vi "SVA 4MV6 P01 CCE RRMA.vi"() -> ()   [LabVIEW 2020]
doc: "Ceballos Conde Emanuel Rodríguez Ramírez Miguel Ángel 4MV6 Sistemas de visión artificial 2022/1\nEste vi permite obtener la distancia en X y Z a la cual se encuentra en objeto u objetos(un maximo de 3 siempre y cuando el color de cada objeto sea de cada una las componentes del sistema rgb) de un sisitema de vision estereoscopico. el usuario puede definir el foco y la distancia del sisitema, a su vez presenta las capturas obtenidas de dichas camara, una representacion en 3d (en el plano XZ) de la escena capturada y permite observar la imagenes binarizadas obtenidas de la descomosicion rgb de cada captura"
uses:
  <vilib>/userDefined/High Color/IMAQdx.ctl
  SVA 4MV6 P01 CCE RRMA.ctl
  <vilib>/vision/driver/IMAQdx.llb/IMAQdx Buffer Number Mode.ctl
  <vilib>/vision/driver/NI_Vision_Acquisition_Software.lvlib
panel:
  in  "umbral\nsuperior":u8=255
  in  "umbral\ninferior":u8=100
  out "Espera":bool
  out "Escena recreada":refnum<vi>(3d-picture)
  in  "Foco\nde la \ncamara":dbl=1331.0
  in  "Distancia\nentre \ncamaras":dbl=20.0 format="%#_13g"
  out "XR":i32
  out "XB":i32
  out "XG":i32
  out "Imagen binaria azul  izquierda":T1(plugin-control)
  out "Imagen binaria verde  izquierda":T1(plugin-control)
  out "Imagen binaria roja  izquierda":T1(plugin-control)
  out "Imagen binaria azul  derecha":T1(plugin-control)
  out "Imagen binaria verde derecha":T1(plugin-control)
  out "Imagen binaria roja  derecha":T1(plugin-control)
  out "ZB":i32
  out "ZG":i32
  out "ZR":i32
  out "Cal Dis":bool
  out "Cap izq":bool
  out "Cap der":bool
  in  "calcular distancia":bool
  in  "capturar imagen izquierda":bool
  in  "capturar Imagen derecha":bool
  out "Imagen izquierda":T1(plugin-control)
  out "Entrada de video":T1(plugin-control)
  in  "stop":bool
  in  "Session In":T2
  out "Imagen derecha":T1(plugin-control)
  # "Controles"
  # "Ceballos Conde Emanuel\nRodríguez Ramírez Miguel Ángel\n4MV6\nSistemas de visión artificial\n2022/1"
  # "Estado"
  # "Resultados en cm"
  # "Configuración"
  # "Binarizado"
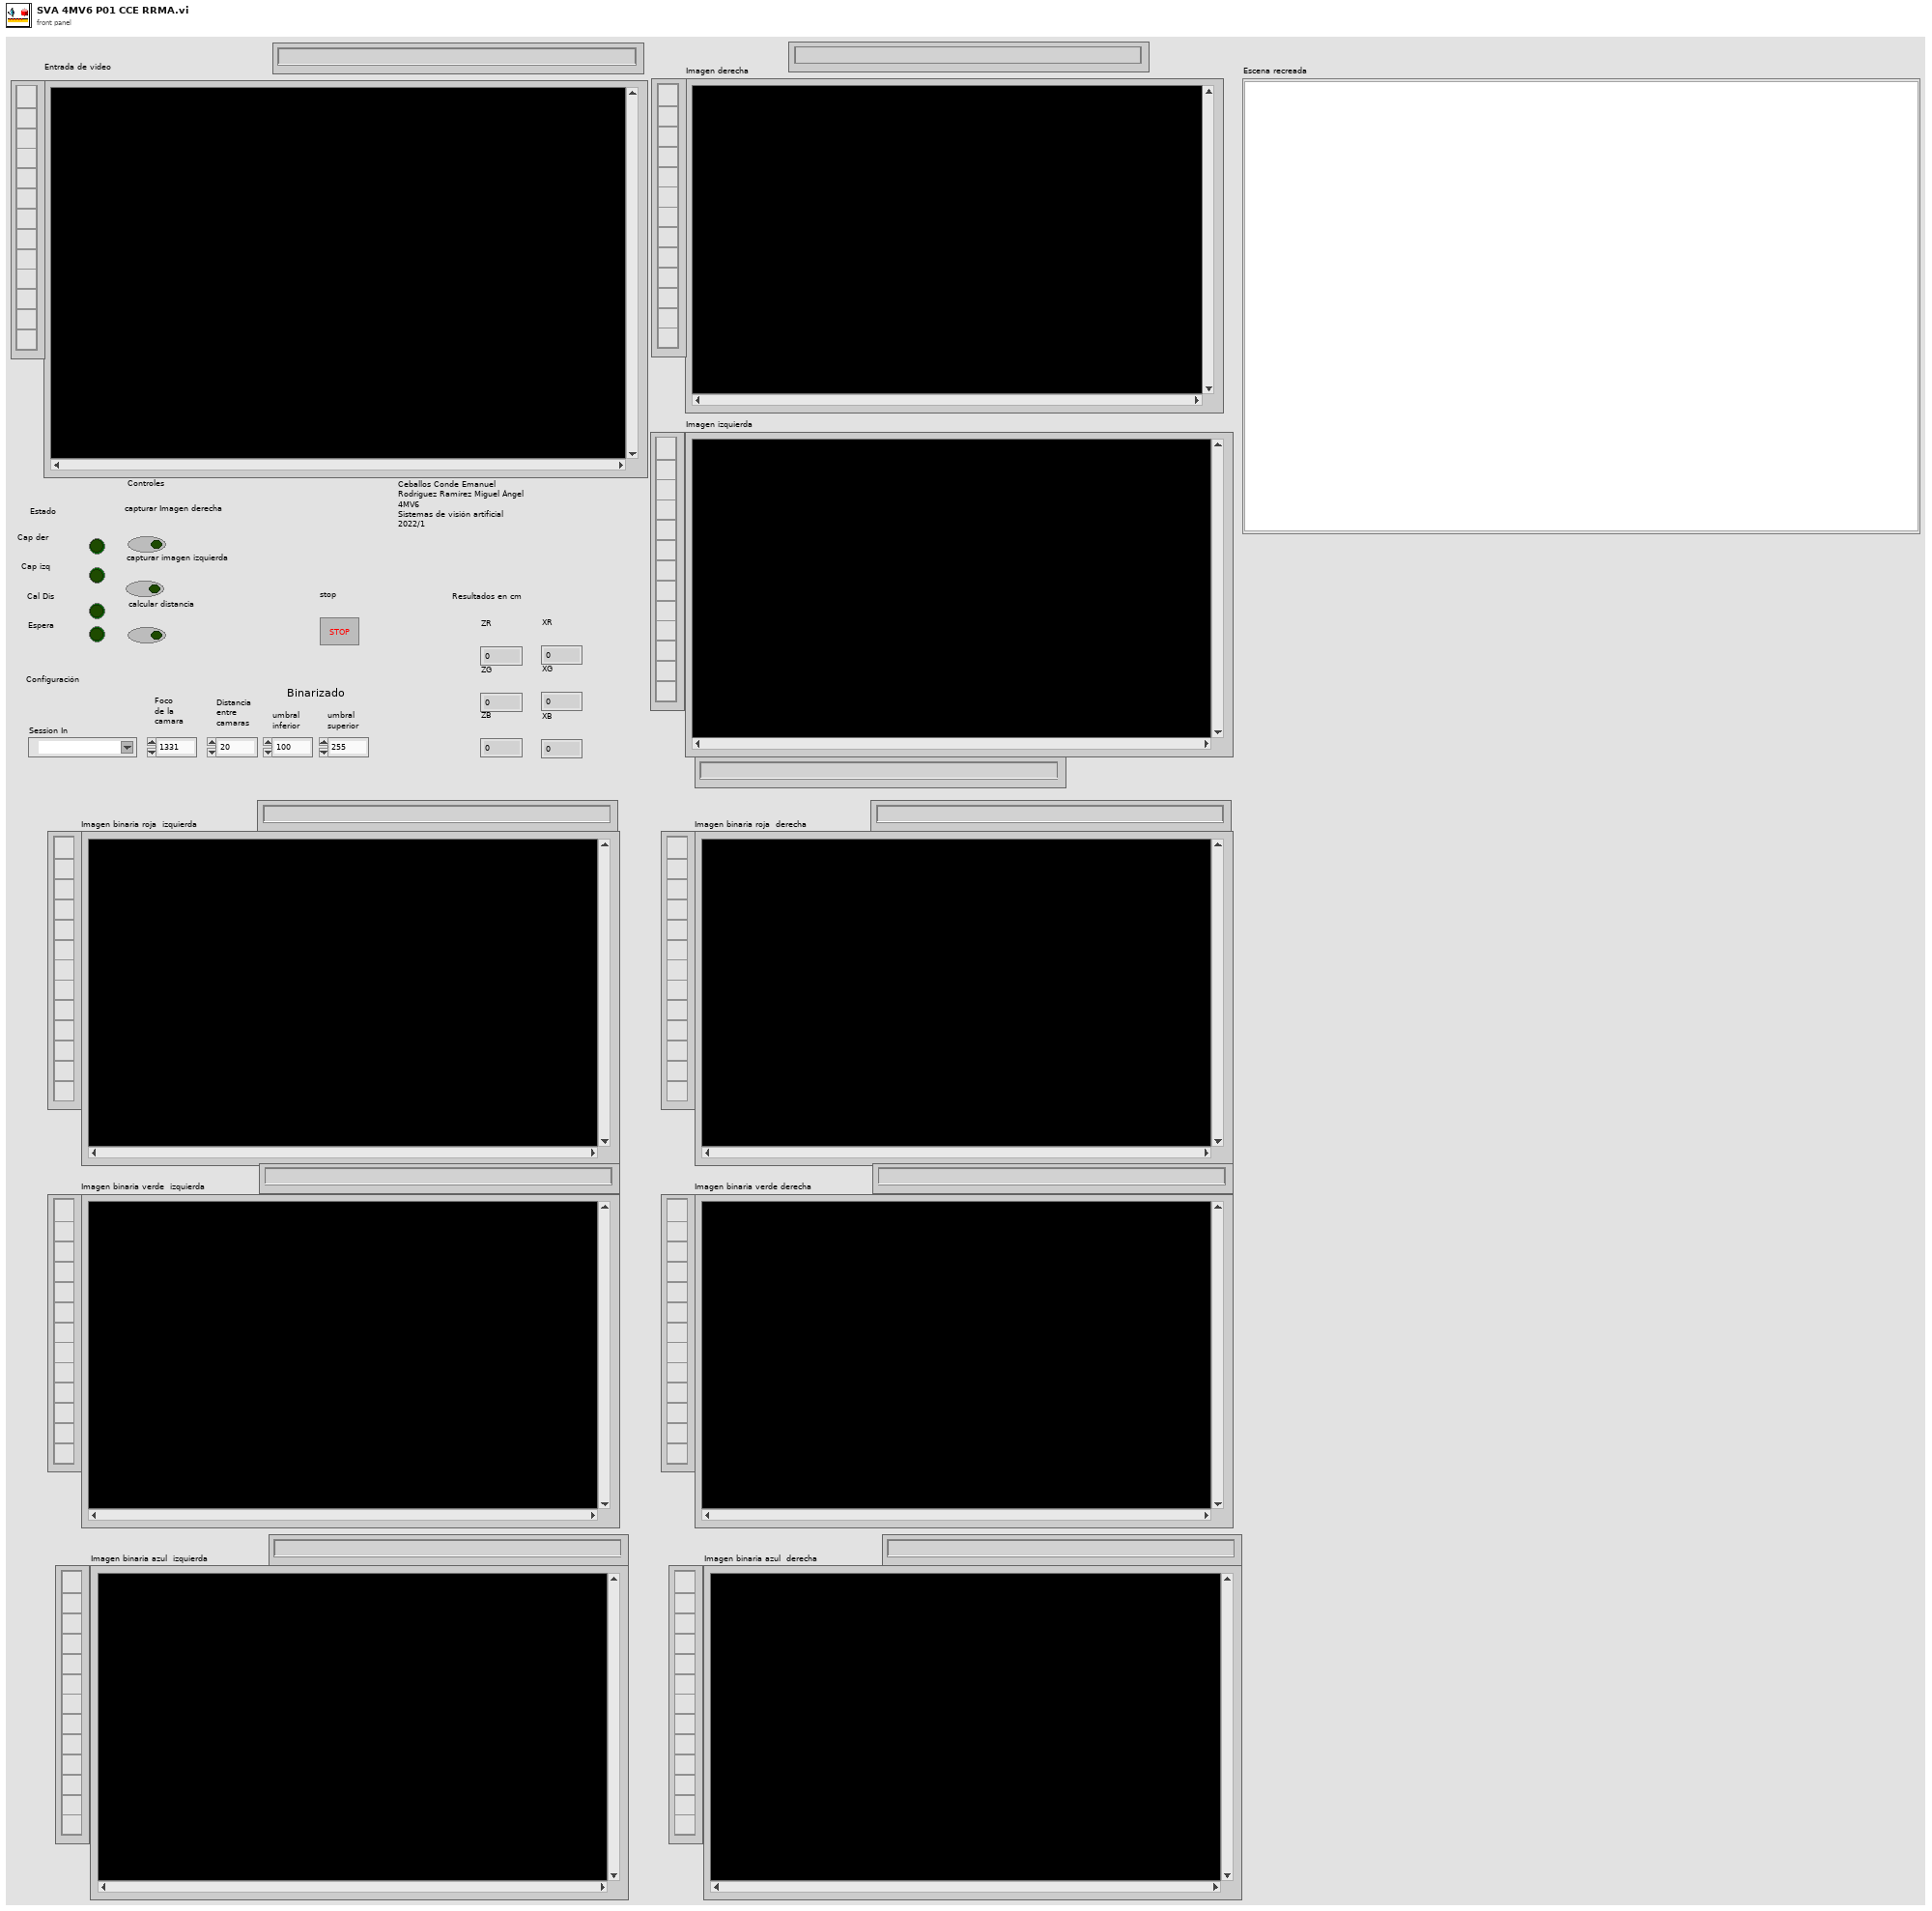
[diagram p1: front panel]
types:
  T1 = typedef "IMAQ Image.ctl" = refnum<image>
  T2 = typedef "IMAQdx.ctl" = refnum<k21>
  T3 = typedef "Image Type" = u32
  T4 = typedef "SVA 4MV6 P01 CCE RRMA.ctl" = enum16{"captura imagen derecha", "captura imagen izquierda", "calculo de distancia", "espera"}
  T5 = typedef "NI_Vision_Acquisition_Software.lvlib/IMAQdx Buffer Number Mode.ctl" = enum32{"Next", "Last", "Buffer Number", "Every", "Last New"}
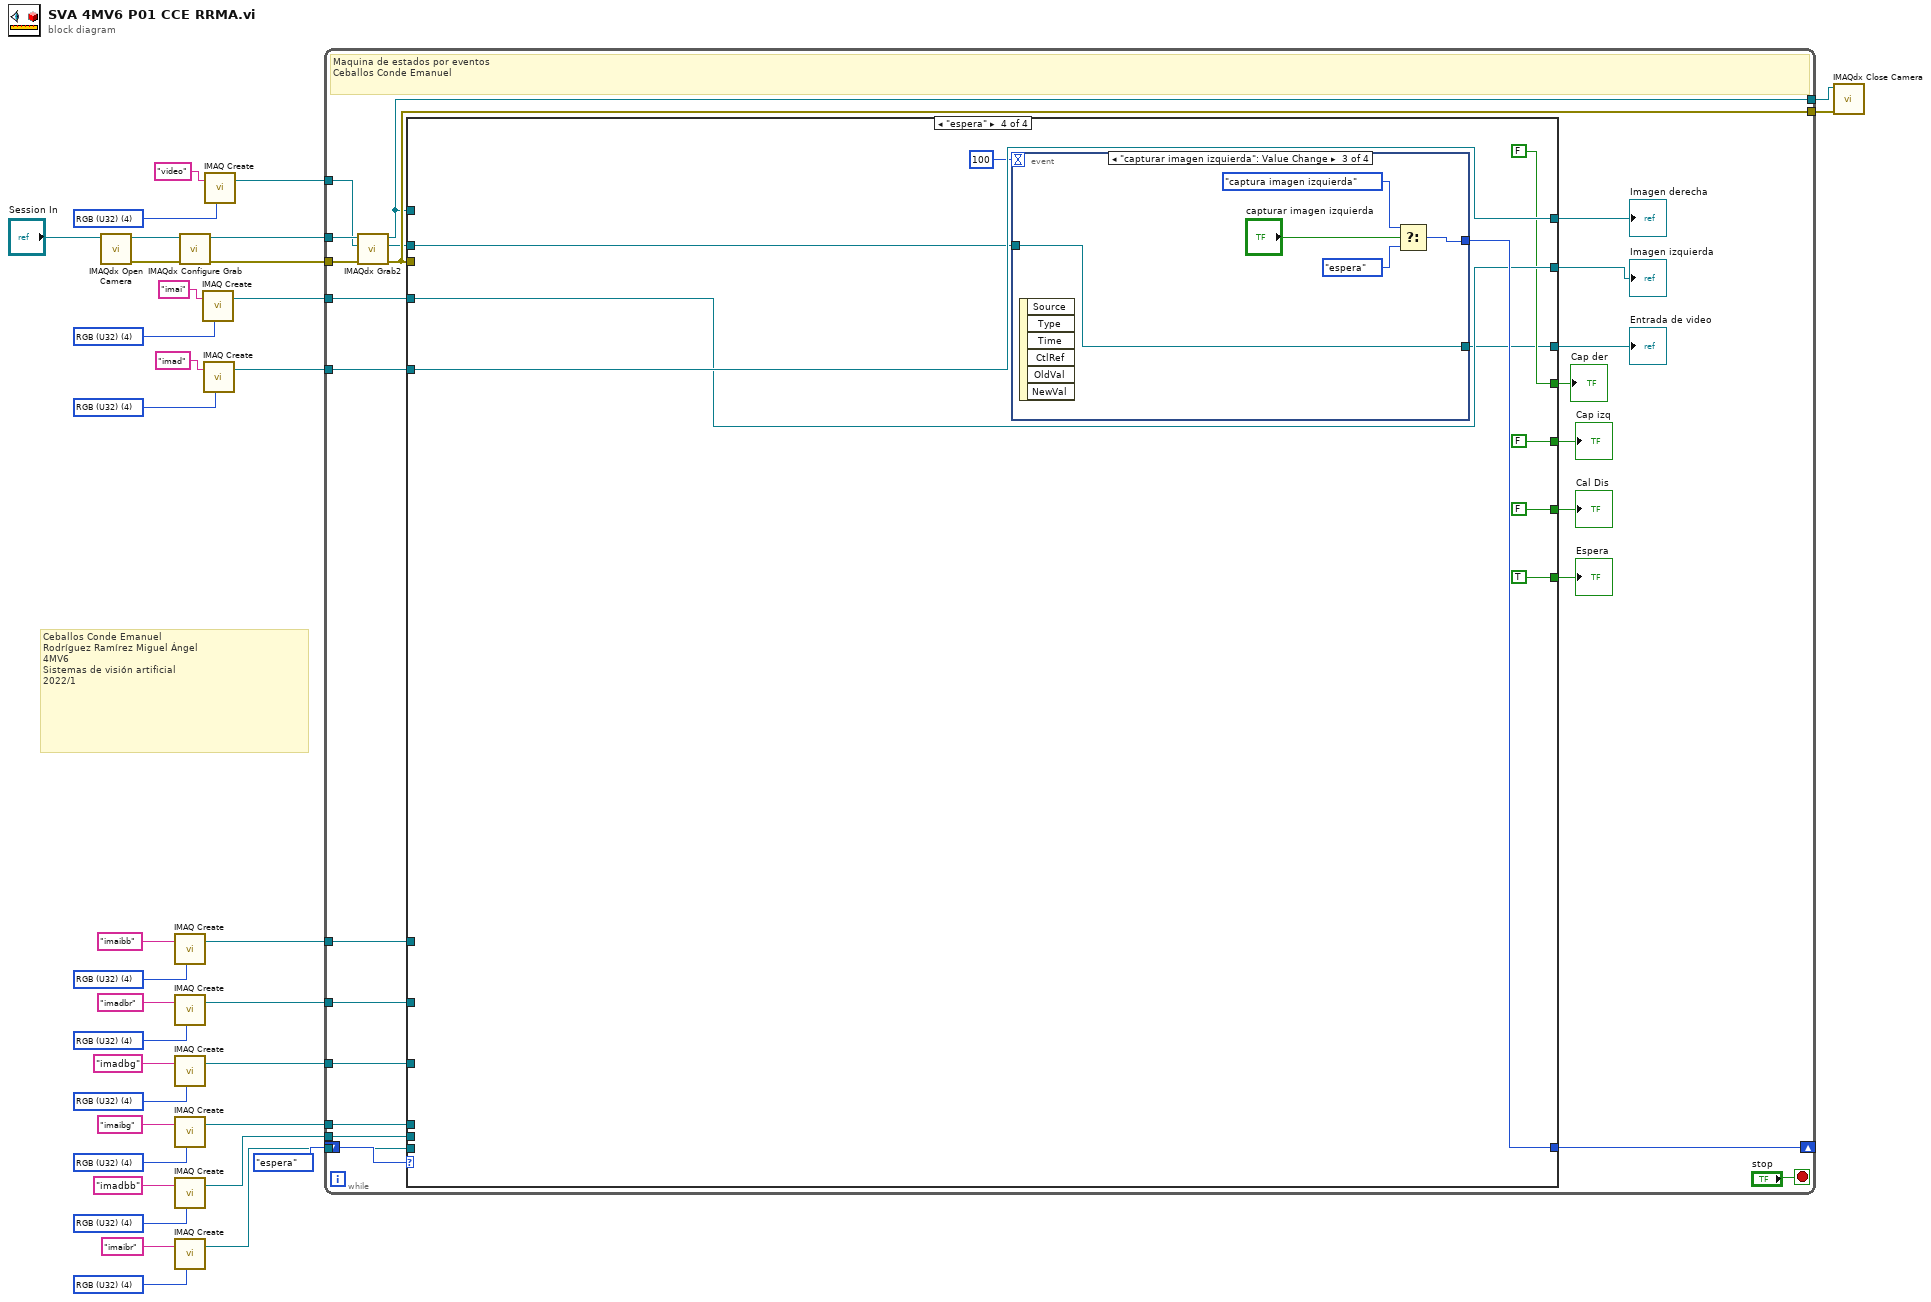
[diagram p0: block diagram]
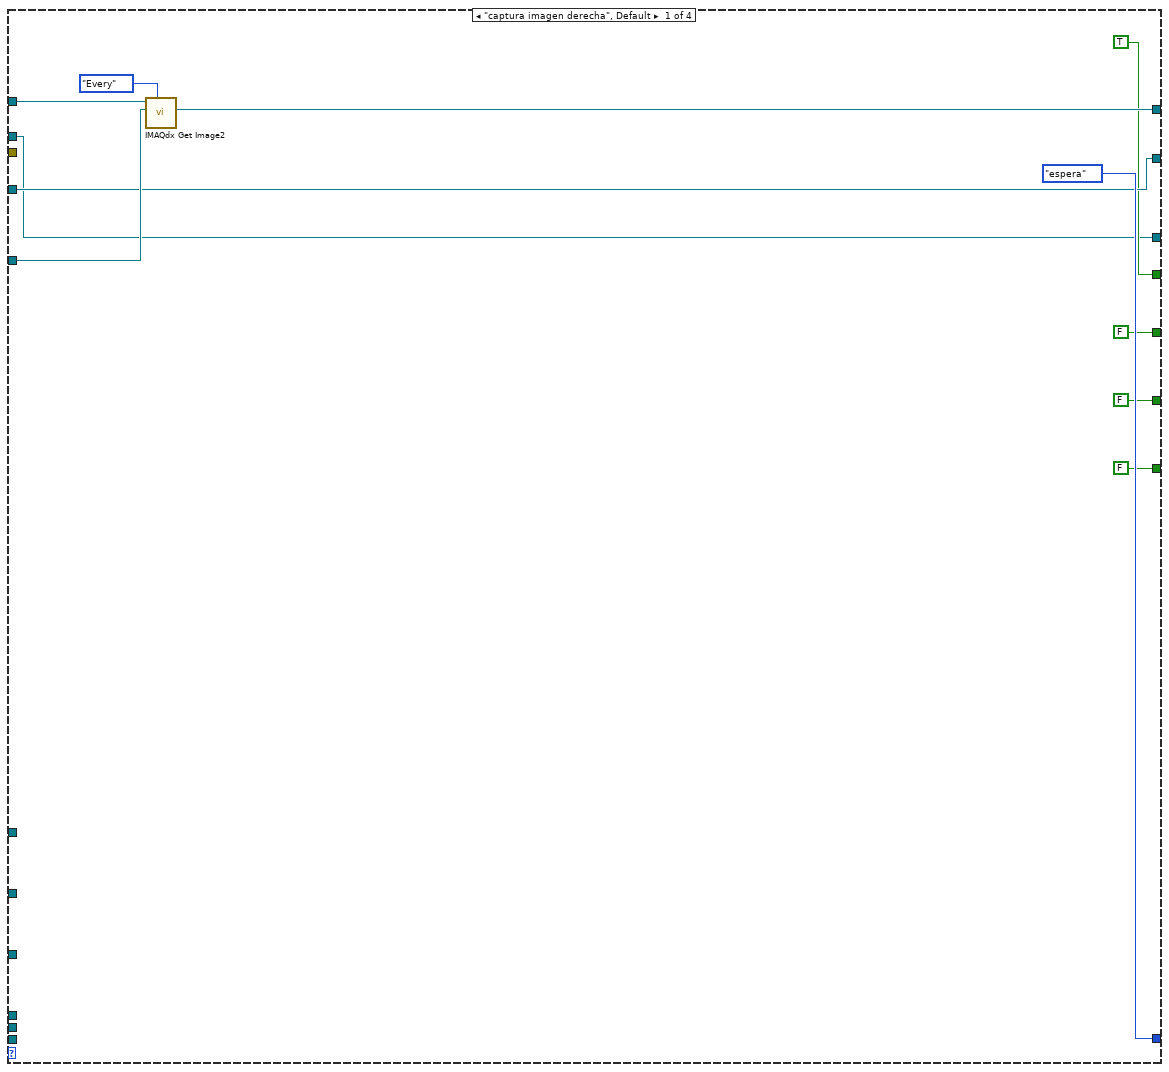
[diagram p2: hidden frame]
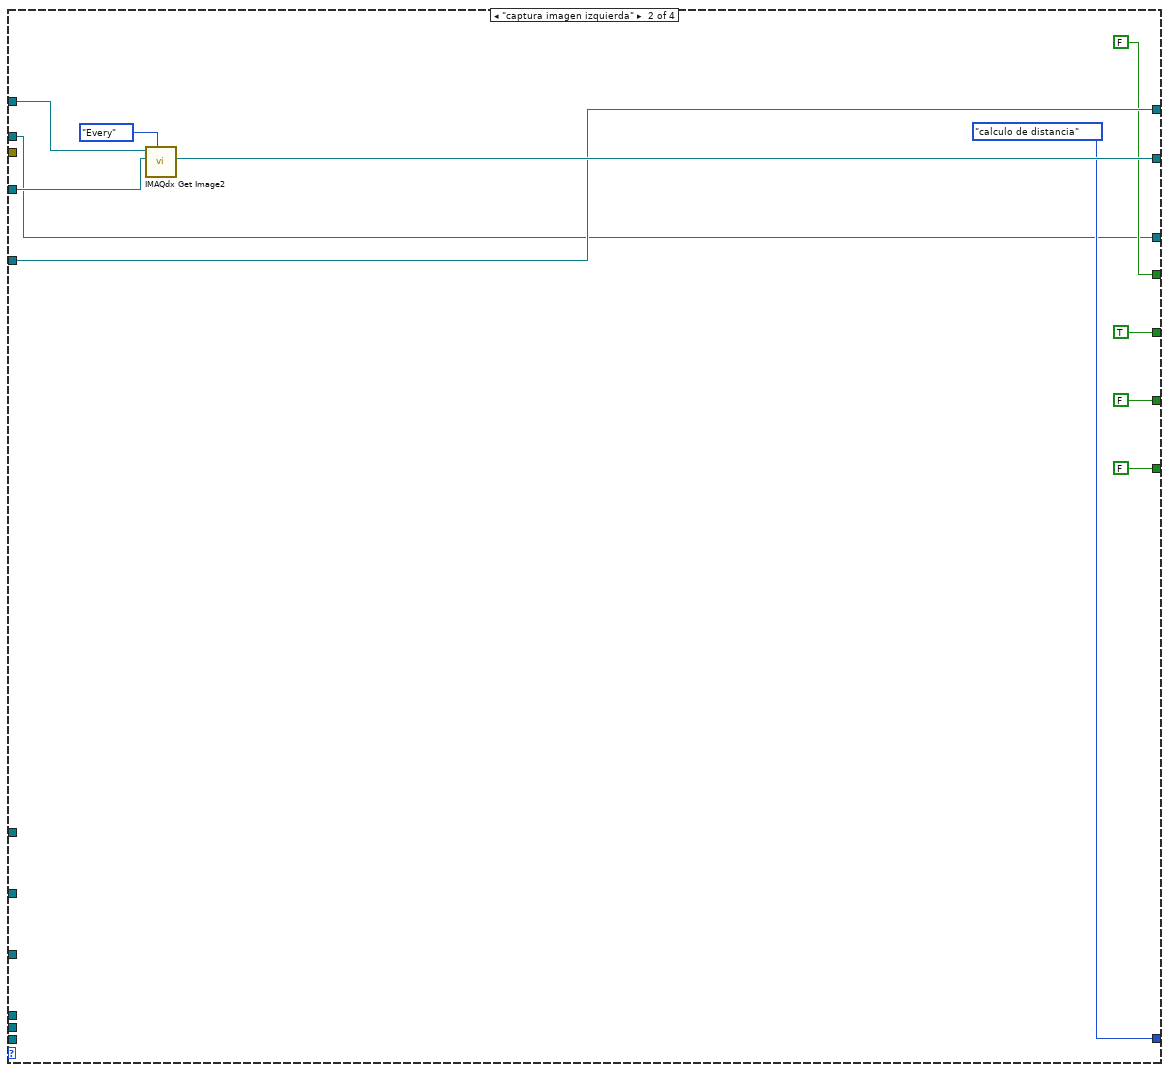
[diagram p3: hidden frame]
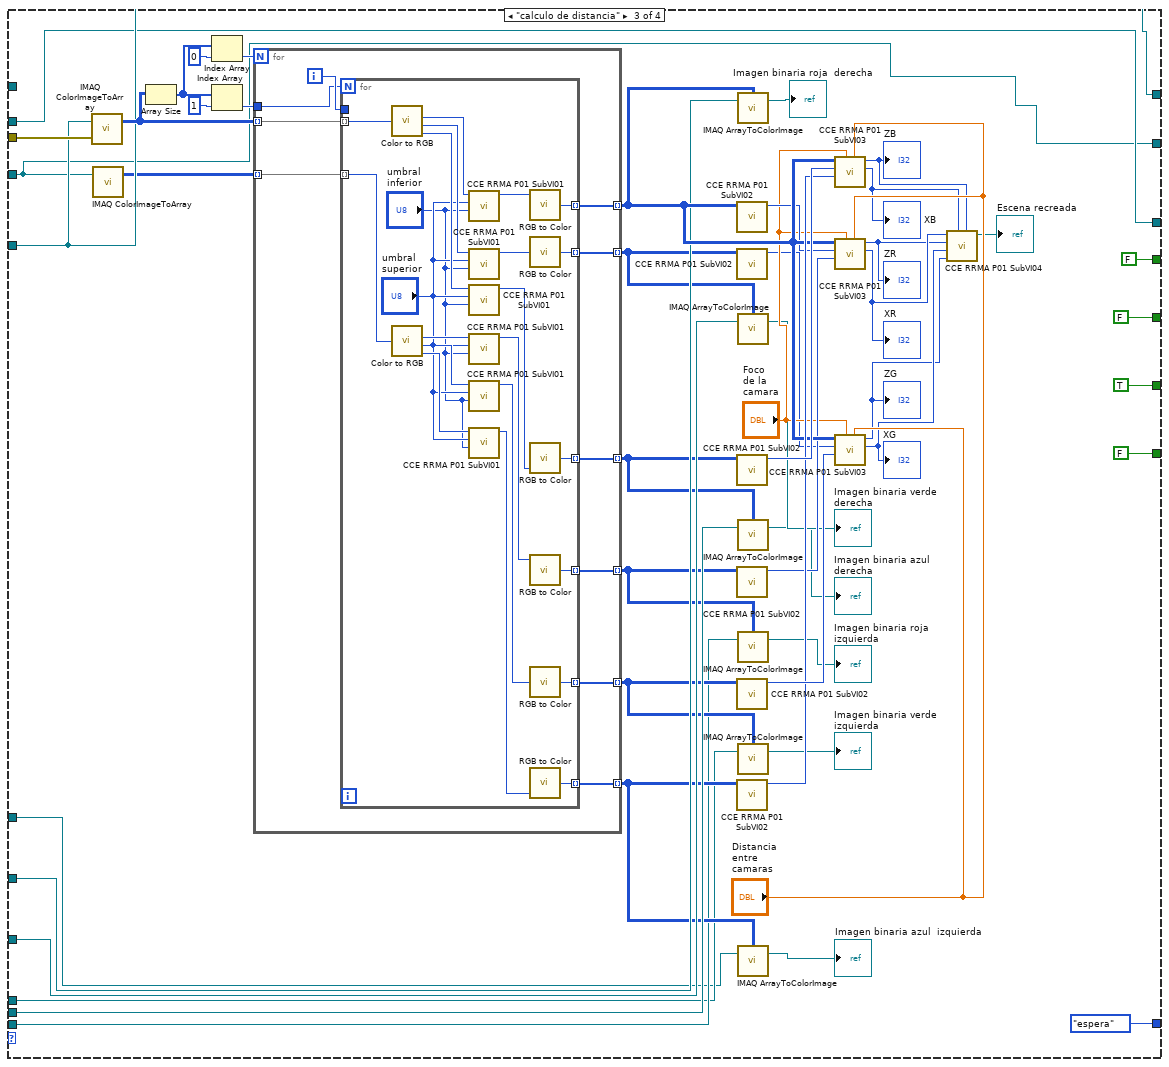
[diagram p4: hidden frame]
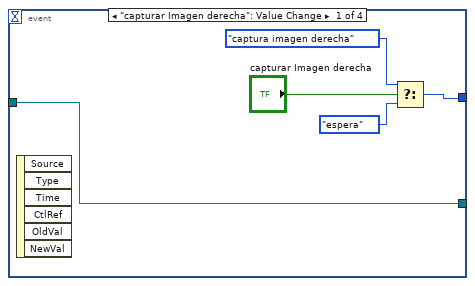
[diagram p5: hidden frame]
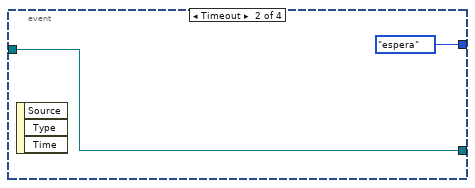
[diagram p6: hidden frame]
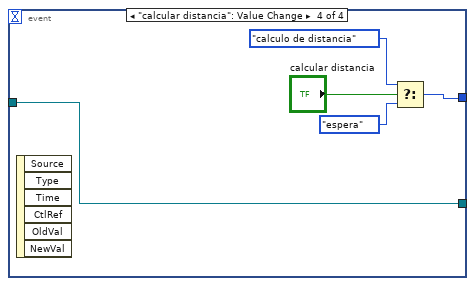
[diagram p7: hidden frame]
diagram:
  w5 = T3 4 items=["Grayscale (U8)", "Grayscale (I16)", "Grayscale (SGL)", "Complex (CSG)", "RGB (U32)", "HSL (U32)", "RGB (U64)", "Grayscale (U16)"] ("Image Type")
  w7 = T3 4 items=["Grayscale (U8)", "Grayscale (I16)", "Grayscale (SGL)", "Complex (CSG)", "RGB (U32)", "HSL (U32)", "RGB (U64)", "Grayscale (U16)"] ("Image Type")
  w9 = T3 4 items=["Grayscale (U8)", "Grayscale (I16)", "Grayscale (SGL)", "Complex (CSG)", "RGB (U32)", "HSL (U32)", "RGB (U64)", "Grayscale (U16)"] ("Image Type")
  w13 = T3 4 items=["Grayscale (U8)", "Grayscale (I16)", "Grayscale (SGL)", "Complex (CSG)", "RGB (U32)", "HSL (U32)", "RGB (U64)", "Grayscale (U16)"] ("Image Type")
  w15 = T3 4 items=["Grayscale (U8)", "Grayscale (I16)", "Grayscale (SGL)", "Complex (CSG)", "RGB (U32)", "HSL (U32)", "RGB (U64)", "Grayscale (U16)"] ("Image Type")
  w18 = T3 4 items=["Grayscale (U8)", "Grayscale (I16)", "Grayscale (SGL)", "Complex (CSG)", "RGB (U32)", "HSL (U32)", "RGB (U64)", "Grayscale (U16)"] ("Image Type")
  w20 = T3 4 items=["Grayscale (U8)", "Grayscale (I16)", "Grayscale (SGL)", "Complex (CSG)", "RGB (U32)", "HSL (U32)", "RGB (U64)", "Grayscale (U16)"] ("Image Type")
  w28 = T3 4 items=["Grayscale (U8)", "Grayscale (I16)", "Grayscale (SGL)", "Complex (CSG)", "RGB (U32)", "HSL (U32)", "RGB (U64)", "Grayscale (U16)"] ("Image Type")
  w33 = T3 4 items=["Grayscale (U8)", "Grayscale (I16)", "Grayscale (SGL)", "Complex (CSG)", "RGB (U32)", "HSL (U32)", "RGB (U64)", "Grayscale (U16)"] ("Image Type")
  # "Ceballos Conde Emanuel\nRodríguez Ramírez Miguel Ángel\n4MV6\nSistemas de visión artificial\n2022/1"
  n1 = call <vilib>:"IMAQdx Open Camera.vi"("Session In"="Session In") -> ("error out"=w31:errorcluster, "Session Out"=w32:T2)  [unwired: 9 in]
  n2 = call "IMAQ Create"("Image Name"="imaibb", "Image Type"=w5) -> ("New Image"=w1:T1)  [unwired: 3 in, 1 out]
  n3 = call "IMAQ Create"("Image Name"="imadbr", "Image Type"=w18) -> ("New Image"=w16:T1)  [unwired: 3 in, 1 out]
  n4 = call "IMAQ Create"("Image Name"="imadbg", "Image Type"=w15) -> ("New Image"=w11:T1)  [unwired: 3 in, 1 out]
  n5 = call "IMAQ Create"("Image Name"="imaibg", "Image Type"=w7) -> ("New Image"=w2:T1)  [unwired: 3 in, 1 out]
  n6 = call "IMAQ Create"("Image Name"="imadbb", "Image Type"=w13) -> ("New Image"=w10:T1)  [unwired: 3 in, 1 out]
  n7 = call "IMAQ Create"("Image Name"="imaibr", "Image Type"=w9) -> ("New Image"=w3:T1)  [unwired: 3 in, 1 out]
  n8 = call <vilib>:"IMAQdx Configure Grab.vi"("error in"=w31, "Session In"=w32) -> ("error out"=w26:errorcluster, "Session Out"=w27:T2)  [unwired: 8 in]
  n9 = call "IMAQ Create"("Image Name"="imai", "Image Type"=w20) -> ("New Image"=w19:T1)  [unwired: 3 in, 1 out]
  n10 = call "IMAQ Create"("Image Name"="imad", "Image Type"=w33) -> ("New Image"=w35:T1)  [unwired: 3 in, 1 out]
  n11 = call "IMAQ Create"("Image Name"="video", "Image Type"=w28) -> ("New Image"=w25:T1)  [unwired: 3 in, 1 out]
  n12 = while {
    tunnel: w27 -> [w59]
    tunnel: w26 -> [w58]
    tunnel: w25 -> [w57]
    tunnel: [w46] -> w24
    tunnel: [w55] -> w23
    shift-right: [w53] -> _
    shift-left: SVA_4MV6_P01_CCE_RRMA."espera" ("Método") -> [w45]
    tunnel: w35 -> [w54]
    tunnel: w19 -> [w52]
    tunnel: w16 -> [w42]
    tunnel: w11 -> [w41]
    tunnel: w10 -> [w40]
    tunnel: w3 -> [w39]
    tunnel: w2 -> [w38]
    tunnel: w1 -> [w37]
    stop <- "stop" stop-if-true
    # "Maquina de estados por eventos\nCeballos Conde Emanuel"
    n13 = call <vilib>:"IMAQdx Grab2.vi"("error in"=w58, "Image In"=w57, "Session In"=w59) -> ("error out"=w55:errorcluster, "Image Out"=w44:T1, "Session Out"=w46:T2)  [unwired: 5 in, 1 out]
    n14 = case shown="\"espera\"" w45 {
      tunnel: w55 -> [_ _ w128 _]
      tunnel: w54 -> [w70 w78 w123 w171]
      tunnel: w46 -> [w68 w80 _ _]
      tunnel: [SVA_4MV6_P01_CCE_RRMA."espera" ("Método") SVA_4MV6_P01_CCE_RRMA."calculo de distancia" ("Método") SVA_4MV6_P01_CCE_RRMA."espera" ("Método") w172] -> w53
      tunnel: w52 -> [w66 w81 w117 w170]
      tunnel: [w67 w78 w123 w171] -> w51
      tunnel: [w66 w79 w117 w170] -> w50
      tunnel: [TRUE ("CID") FALSE ("CID") FALSE ("CID") FALSE ("CID")] -> w49
      tunnel: [FALSE ("CID") TRUE ("CID") FALSE ("CID") FALSE ("CID")] -> w48
      tunnel: [FALSE ("CID") FALSE ("CID") TRUE ("CID") FALSE ("CID")] -> w47
      tunnel: w44 -> [w61 w72 w118 w166]
      tunnel: [w61 w72 w118 w165] -> w43
      tunnel: w42 -> [_ _ w109 _]
      tunnel: w41 -> [_ _ w103 _]
      tunnel: w40 -> [_ _ w102 _]
      tunnel: w39 -> [_ _ w93 _]
      tunnel: w38 -> [_ _ w92 _]
      tunnel: w37 -> [_ _ w91 _]
      tunnel: [FALSE ("CID") FALSE ("CID") FALSE ("CID") TRUE ("CID")] -> w36
      frame "captura imagen derecha", Default {
        n15 = call <vilib>:"IMAQdx Get Image2.vi"("Buffer Number Mode (Next)"=IMAQdx_Buffer_Number_Mode."Every", "Image In"=w70, "Session In"=w68) -> ("Image Out"=w67:T1)  [unwired: 5 in, 3 out]
      }
      frame "captura imagen izquierda" {
        n16 = call <vilib>:"IMAQdx Get Image2.vi"("Buffer Number Mode (Next)"=IMAQdx_Buffer_Number_Mode."Every", "Image In"=w81, "Session In"=w80) -> ("Image Out"=w79:T1)  [unwired: 5 in, 3 out]
      }
      frame "calculo de distancia" {
        n17 = call "IMAQ ColorImageToArray"("Image"=w123, "error in (no error)"=w128) -> ("Image Pixels (U32)"=w129:u32[][])  [unwired: 2 in, 2 out]
        n18 = call "IMAQ ColorImageToArray"("Image"=w117) -> ("Image Pixels (U32)"=w116:u32[][])  [unwired: 3 in, 2 out]
        n19 = Array Size(array=w129) -> (size(s)=w130:i32[])
        n20 = Index Array(array=w130, index=0) -> (element=w127:i32)
        n21 = Index Array(array=w130, index=1) -> (element=w125:i32)
        n22 = for {
          N: w127 -> [_]
          tunnel: w129 -> [w140] mode=indexing
          tunnel: [w138] -> w110 mode=indexing
          tunnel: w125 -> [w137]
          tunnel: [w136] -> w101 mode=indexing
          tunnel: [w135] -> w100 mode=indexing
          tunnel: w116 -> [w134] mode=indexing
          tunnel: [w133] -> w96 mode=indexing
          tunnel: [w132] -> w95 mode=indexing
          tunnel: [w131] -> w94 mode=indexing
          i -> [w139]
          n23 = for {
            N: w137 -> [_]
            tunnel: w140 -> [w162] mode=indexing
            tunnel: w139 -> [_]
            tunnel: [w157] -> w138 mode=indexing
            tunnel: [w154] -> w136 mode=indexing
            tunnel: [w153] -> w135 mode=indexing
            tunnel: w134 -> [w146] mode=indexing
            tunnel: [w145] -> w133 mode=indexing
            tunnel: [w144] -> w132 mode=indexing
            tunnel: [w143] -> w131 mode=indexing
            n24 = call <vilib>:"Color to RGB.vi"("Color"=w162) -> ("R"=w159:u8, "G"=w160:u8, "B"=w161:u8)  [unwired: 1 out]
            n25 = call <vilib>:"Color to RGB.vi"("Color"=w146) -> ("R"=w150:u8, "G"=w151:u8, "B"=w152:u8)  [unwired: 1 out]
            n26 = call "CCE RRMA P01 SubVI01.vi"("imagen"=w159, "umbral superior"="umbral\nsuperior", "umbral inferior"="umbral\ninferior") -> ("umbralizado"=w158:u8)  [unwired: 7 in]
            n27 = call "CCE RRMA P01 SubVI01.vi"("imagen"=w160, "umbral superior"="umbral\nsuperior", "umbral inferior"="umbral\ninferior") -> ("umbralizado"=w156:u8)  [unwired: 7 in]
            n28 = call "CCE RRMA P01 SubVI01.vi"("imagen"=w161, "umbral superior"="umbral\nsuperior", "umbral inferior"="umbral\ninferior") -> ("umbralizado"=w155:u8)  [unwired: 7 in]
            n29 = call "CCE RRMA P01 SubVI01.vi"("imagen"=w150, "umbral superior"="umbral\nsuperior", "umbral inferior"="umbral\ninferior") -> ("umbralizado"=w149:u8)  [unwired: 7 in]
            n30 = call "CCE RRMA P01 SubVI01.vi"("imagen"=w151, "umbral superior"="umbral\nsuperior", "umbral inferior"="umbral\ninferior") -> ("umbralizado"=w148:u8)  [unwired: 7 in]
            n31 = call "CCE RRMA P01 SubVI01.vi"("imagen"=w152, "umbral superior"="umbral\nsuperior", "umbral inferior"="umbral\ninferior") -> ("umbralizado"=w147:u8)  [unwired: 7 in]
            n32 = call <vilib>:"RGB to Color.vi"("R"=w158) -> ("Color"=w157:u32)  [unwired: 2 in]
            n33 = call <vilib>:"RGB to Color.vi"("G"=w156) -> ("Color"=w154:u32)  [unwired: 2 in]
            n34 = call <vilib>:"RGB to Color.vi"("B"=w155) -> ("Color"=w153:u32)  [unwired: 2 in]
            n35 = call <vilib>:"RGB to Color.vi"("R"=w149) -> ("Color"=w145:u32)  [unwired: 2 in]
            n36 = call <vilib>:"RGB to Color.vi"("G"=w148) -> ("Color"=w144:u32)  [unwired: 2 in]
            n37 = call <vilib>:"RGB to Color.vi"("B"=w147) -> ("Color"=w143:u32)  [unwired: 2 in]
          }
        }
        n38 = call "CCE RRMA P01 SubVI02.vi"("Array"=w110) -> ("cx"=w108:u32)  [unwired: 9 in, 1 out]
        n39 = call "CCE RRMA P01 SubVI02.vi"("Array"=w101) -> ("cx"=w83:u32)  [unwired: 9 in, 1 out]
        n40 = call "CCE RRMA P01 SubVI02.vi"("Array"=w100) -> ("cx"=w113:u32)  [unwired: 9 in, 1 out]
        n41 = call "CCE RRMA P01 SubVI02.vi"("Array"=w96) -> ("cx"=w107:u32)  [unwired: 9 in, 1 out]
        n42 = call "CCE RRMA P01 SubVI02.vi"("Array"=w95) -> ("cx"=w114:u32)  [unwired: 9 in, 1 out]
        n43 = call "CCE RRMA P01 SubVI02.vi"("Array"=w94) -> ("cx"=w112:u32)  [unwired: 9 in, 1 out]
        n44 = call "IMAQ ArrayToColorImage"("Image Pixels (U32)"=w110, "Image"=w109) -> ("Image Out"=→"Imagen binaria roja  derecha":T1)  [unwired: 3 in, 1 out]
        n45 = call "IMAQ ArrayToColorImage"("Image Pixels (U32)"=w101, "Image"=w103) -> ("Image Out"=→"Imagen binaria verde derecha":T1)  [unwired: 3 in, 1 out]
        n46 = call "IMAQ ArrayToColorImage"("Image Pixels (U32)"=w100, "Image"=w102) -> ("Image Out"=→"Imagen binaria azul  derecha":T1)  [unwired: 3 in, 1 out]
        n47 = call "IMAQ ArrayToColorImage"("Image Pixels (U32)"=w96, "Image"=w93) -> ("Image Out"=→"Imagen binaria roja  izquierda":T1)  [unwired: 3 in, 1 out]
        n48 = call "IMAQ ArrayToColorImage"("Image Pixels (U32)"=w95, "Image"=w92) -> ("Image Out"=→"Imagen binaria verde  izquierda":T1)  [unwired: 3 in, 1 out]
        n49 = call "IMAQ ArrayToColorImage"("Image Pixels (U32)"=w94, "Image"=w91) -> ("Image Out"=→"Imagen binaria azul  izquierda":T1)  [unwired: 3 in, 1 out]
        n50 = call "CCE RRMA P01 SubVI03.vi"("d"="Distancia\nentre \ncamaras", "f"="Foco\nde la \ncamara", "xi"=w112, "xd"=w113, "array"=w110) -> ("X"=w86:i32, "Z"=w85:i32)  [unwired: 5 in]
        "ZB" <- w85
        "XB" <- w86
        n51 = call "CCE RRMA P01 SubVI03.vi"("d"="Distancia\nentre \ncamaras", "f"="Foco\nde la \ncamara", "xi"=w107, "xd"=w108, "array"=w110) -> ("X"=w90:i32, "Z"=w89:i32)  [unwired: 5 in]
        "ZR" <- w89
        "XR" <- w90
        n52 = call "CCE RRMA P01 SubVI03.vi"("d"="Distancia\nentre \ncamaras", "f"="Foco\nde la \ncamara", "xi"=w114, "xd"=w83, "array"=w110) -> ("X"=w88:i32, "Z"=w87:i32)  [unwired: 5 in]
        "ZG" <- w87
        "XG" <- w88
        n53 = call "CCE RRMA P01 SubVI04.vi"("ZB"=w85, "XB"=w86, "ZG"=w87, "XG"=w88, "ZR"=w89, "XR"=w90) -> ("3D Picture"=→"Escena recreada":refnum<vi>)  [unwired: 5 in]
      }
      frame "espera" {
        n54 = event shown="[2] \"capturar imagen izquierda\": Value Change" {
          selector: _ -> [_ _ _ _]
          dyn-events: _ -> [_ _ _ _]
          timeout: 100 -> [_ _ _ _]
          tunnel: [w174 SVA_4MV6_P01_CCE_RRMA."espera" ("Método") w181 w186] -> w172
          tunnel: w166 -> [w173 w178 w180 w185]
          tunnel: [w173 w178 w180 w185] -> w165
          event "capturar Imagen derecha": Value Change {
            n55 = event-data() -> ()  [unwired: 1 in, 6 out]
            n56 = Select(t=SVA_4MV6_P01_CCE_RRMA."captura imagen derecha" ("Método"), s="capturar Imagen derecha", f=SVA_4MV6_P01_CCE_RRMA."espera" ("Método")) -> (s? t:f=w174:T4)
          }
          event Timeout {
            n57 = event-data() -> ()  [unwired: 1 in, 3 out]
          }
          event "capturar imagen izquierda": Value Change {
            n58 = event-data() -> ()  [unwired: 1 in, 6 out]
            n59 = Select(t=SVA_4MV6_P01_CCE_RRMA."captura imagen izquierda" ("Método"), s="capturar imagen izquierda", f=SVA_4MV6_P01_CCE_RRMA."espera" ("Método")) -> (s? t:f=w181:T4)
          }
          event "calcular distancia": Value Change {
            n60 = event-data() -> ()  [unwired: 1 in, 6 out]
            n61 = Select(t=SVA_4MV6_P01_CCE_RRMA."calculo de distancia" ("Método"), s="calcular distancia", f=SVA_4MV6_P01_CCE_RRMA."espera" ("Método")) -> (s? t:f=w186:T4)
          }
        }
      }
    }
    "Imagen derecha" <- w51
    "Imagen izquierda" <- w50
    "Cap der" <- w49
    "Cal Dis" <- w47
    "Cap izq" <- w48
    "Entrada de video" <- w43
    "Espera" <- w36
  }
  n62 = call <vilib>:"IMAQdx Close Camera.vi"("error in"=w23, "Session In"=w24) -> ()  [unwired: 9 in, 1 out]
